vi "ModuleUI.vi"() -> ()   [LabVIEW 2013, in "PL Framework Configuration Tool.lvlib" / "module editor node.lvclass"]
uses:
  module editor node.lvclass
  <vilib>/NI/CEF/CEF_TreeControl/Node/NodeRef.ctl
  <vilib>/NI/CEF/CEF_TreeControl/Node/NISE_CEF_Node.lvclass
  <vilib>/NI/AMC/Message Queue.ctl
  <vilib>/NI/AMC/Message.ctl
  <vilib>/NI/Tools/Keyed Array/KeyedArray.ctl
  <vilib>/NI/CEF/CEF_TreeControl/Node/UserEventRef.ctl
  <vilib>/NI/CEF/CEF_TreeControl/Controls/EventCluster.ctl
  <vilib>/NI/Tools/Keyed Array/Tools_KeyedArray.lvlib
  <vilib>/NI/AMC/AMC.lvlib
  <vilib>/NI/CEF/CEF_TreeControl/NISE_CEF_TreeControl.lvlib
panel:
  in  "user event":T1
  in  "main queue":T2
  in  "node ref":T3
  # "node UI"
  # "An error has occurred\n\nThis UI was loaded by a module but it is invalid"
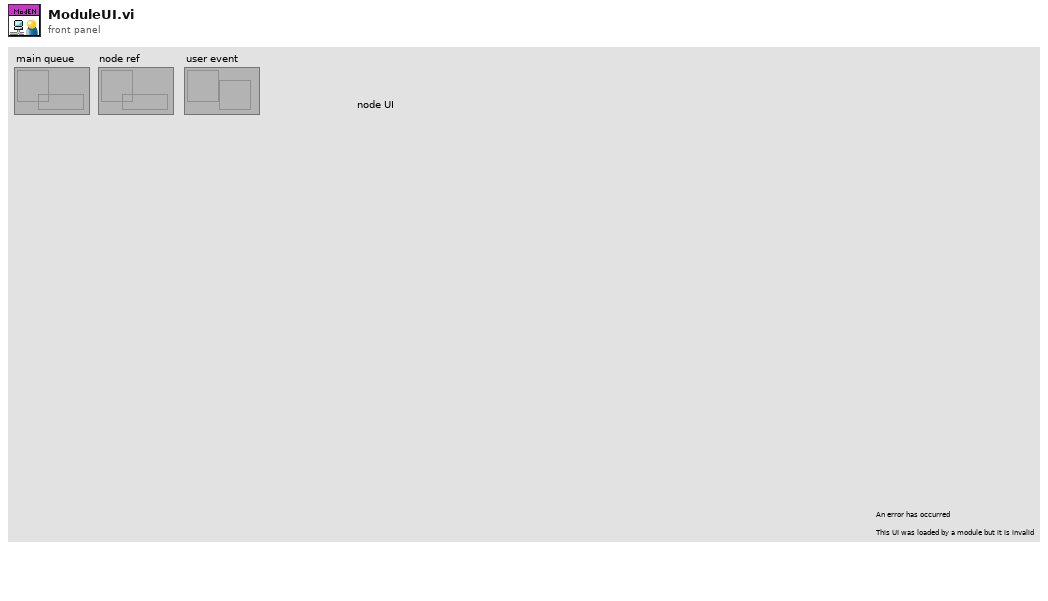
[diagram p1: front panel]
types:
  T1 = typedef "NISE_CEF_Node.lvclass/UserEventRef.ctl" = refnum<user-event>
  T2 = typedef "AMC.lvlib/Message Queue.ctl" = refnum<queue>
  T3 = typedef "NISE_CEF_Node.lvclass/NodeRef.ctl" = refnum<data-value>
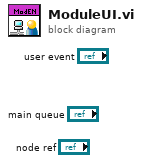
[diagram p0: block diagram]
diagram:
